vi "VA_Averaging_AI.vi"(1 "AnalogIn":dbl[][](array[numeric])) -> (0 "Anolog XYZ":dbl[](array[numeric]))   [LabVIEW 2011]
uses:
  <vilib>/Analysis/NI_AALBase.lvlib
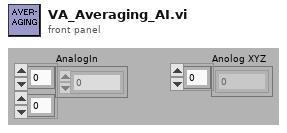
[diagram p1: front panel]
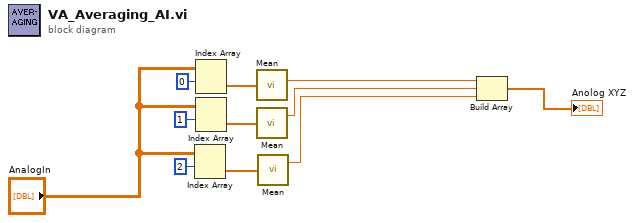
[diagram p0: block diagram]
diagram:
  n1 = Index Array(array="AnalogIn", index (row)=2 ("index")) -> (element=w7:dbl[])  [unwired: 1 in]
  n2 = Index Array(array="AnalogIn", index (row)=0 ("index")) -> (element=w5:dbl[])  [unwired: 1 in]
  n3 = Index Array(array="AnalogIn", index (row)=1 ("index")) -> (element=w6:dbl[])  [unwired: 1 in]
  n4 = call <vilib>:"Mean.vi"("X"=w5) -> ("mean"=w8:dbl)  [unwired: 1 out]
  n5 = call <vilib>:"Mean.vi"("X"=w6) -> ("mean"=w9:dbl)  [unwired: 1 out]
  n6 = call <vilib>:"Mean.vi"("X"=w7) -> ("mean"=w10:dbl)  [unwired: 1 out]
  n7 = Build Array(w8, w9, w10) -> (→"Anolog XYZ":dbl[])
